vi "Get Error Correction Factors.vi"(0 "instrument handle":refnum<k15>, 11 "Error In":errorcluster) -> (4 "instrument handle out":refnum<k15>, 8 "Two Port Correction Factors":T1, 15 "Error Out":errorcluster)   [LabVIEW 2013]
uses:
  Two Port Corerction Factors.ctl
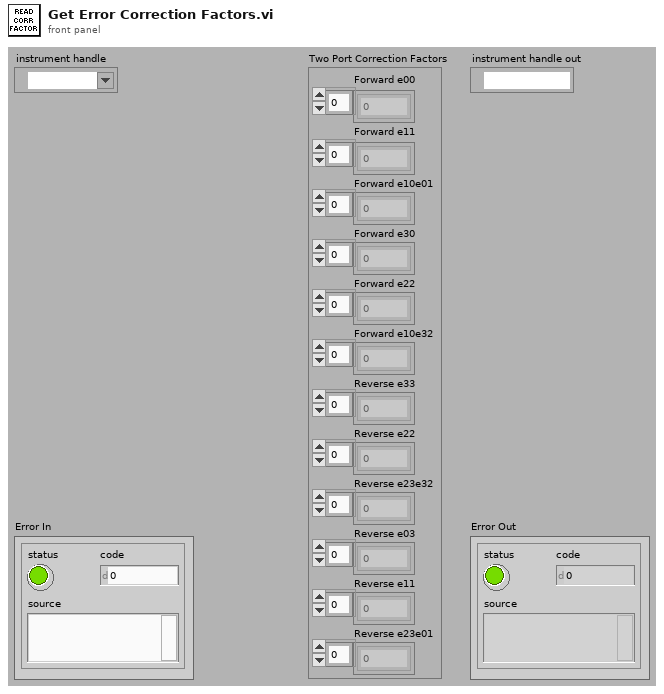
[diagram p1: front panel]
types:
  T1 = typedef "Two Port Corerction Factors.ctl" = cluster{"Forward e00":cdb[], "Forward e11":cdb[], "Forward e10e01":cdb[], "Forward e30":cdb[], "Forward e22":cdb[], "Forward e10e32":cdb[], "Reverse e33":cdb[], "Reverse e22 ":cdb[], "Reverse e23e32":cdb[], "Reverse e03":cdb[], "Reverse e11":cdb[], "Reverse e23e01":cdb[]}
  T2 = enum16{"e00", "e11", "e10e01", "e10e32", "e22", "e30", "e'33", "e'22", "e'23e'32", "e'23e'01", "e'11", "e'03"}[]
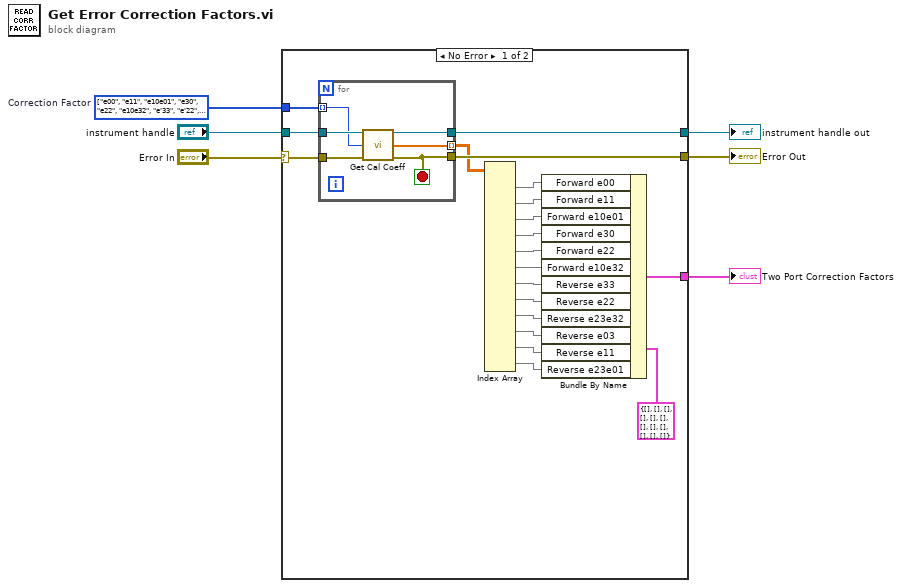
[diagram p0: block diagram]
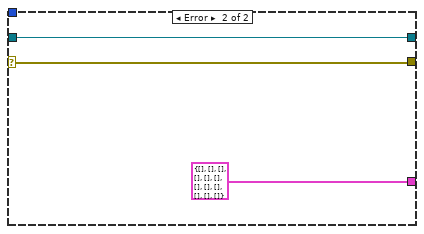
[diagram p2: hidden frame]
diagram:
  w2 = T2 [enum."e00", enum."e11", enum."e10e01", enum."e30", enum."e22", enum."e10e32", enum."e'33", enum."e'22", enum."e'23e'32", enum."e'03", enum."e'11", enum."e'23e'01"] items=["e00", "e11", "e10e01", "e10e32", "e22", "e30", "e'33", "e'22", "e'23e'32", "e'23e'01", "e'11", "e'03"]  # Correction Factor
  n1 = case shown="No Error" "Error In" {
    selector: "Error In" -> [w8 w35]
    tunnel: [w26 w34] -> w6
    tunnel: "instrument handle" -> [w25 w34]
    tunnel: [w24 w35] -> w4
    tunnel: [w10 T1 {"Forward e00"=[], "Forward e11"=[], "Forward e10e01"=[], "Forward e30"=[], "Forward e22"=[], "Forward e10e32"=[], "Reverse e33"=[], "Reverse e22 "=[], "Reverse e23e32"=[], "Reverse e03"=[], "Reverse e11"=[], "Reverse e23e01"=[]} ("Cluster")] -> w3
    tunnel: w2 -> [w9 _]
    frame No Error {
      n2 = for {
        tunnel: w25 -> [w32]
        tunnel: w8 -> [w31]
        tunnel: [w30] -> w26
        tunnel: [w29] -> w24
        tunnel: w9 -> [w28] mode=indexing
        tunnel: [w27] -> w7 mode=indexing
        stop <- w29 stop-if-true
        n3 = call "Get Cal Coeff.vi"("instrument handle"=w32, "Correction Factor"=w28, "Error In"=w31) -> ("instrument handle out"=w30:refnum<k15>, "Correction Factor Array"=w27:csg[], "Error Out"=w29:errorcluster)  [unwired: 10 in]
      }
      n4 = Index Array(array=w7) -> (element #1=w22:csg[], element #2=w21:csg[], element #3=w20:csg[], element #4=w19:csg[], element #5=w18:csg[], element #6=w17:csg[], element #7=w16:csg[], element #8=w15:csg[], element #9=w14:csg[], element #10=w13:csg[], element #11=w12:csg[], element #12=w11:csg[])  [unwired: 24 in]
      n5 = Bundle By Name(cluster=T1 {"Forward e00"=[], "Forward e11"=[], "Forward e10e01"=[], "Forward e30"=[], "Forward e22"=[], "Forward e10e32"=[], "Reverse e33"=[], "Reverse e22 "=[], "Reverse e23e32"=[], "Reverse e03"=[], "Reverse e11"=[], "Reverse e23e01"=[]} ("Cluster"), "Forward e00"=w22, "Forward e11"=w21, "Forward e10e01"=w20, "Forward e30"=w19, "Forward e22"=w18, "Forward e10e32"=w17, "Reverse e33"=w16, "Reverse e22"=w15, "Reverse e23e32"=w14, "Reverse e03"=w13, "Reverse e11"=w12, "Reverse e23e01"=w11) -> (w10:T1)
    }
    frame Error {
    }
  }
  "instrument handle out" <- w6
  "Error Out" <- w4
  "Two Port Correction Factors" <- w3
